vi "Read Instrument Descriptor.vi"(8 "error in (no error)":errorcluster, 11 "PXI 4070 in":refnum<class "PXI 4070.lvclass">) -> (0 "error out":errorcluster, 2 "Instrument Descriptor":refnum<k15>="Dev1", 3 "PXI 4070 out":refnum<class "PXI 4070.lvclass">)   [LabVIEW 2013, in "PXI 4070.lvclass"]
uses:
  PXI 4070.lvclass
  PXI 4070.lvclass/PXI 4070.ctl
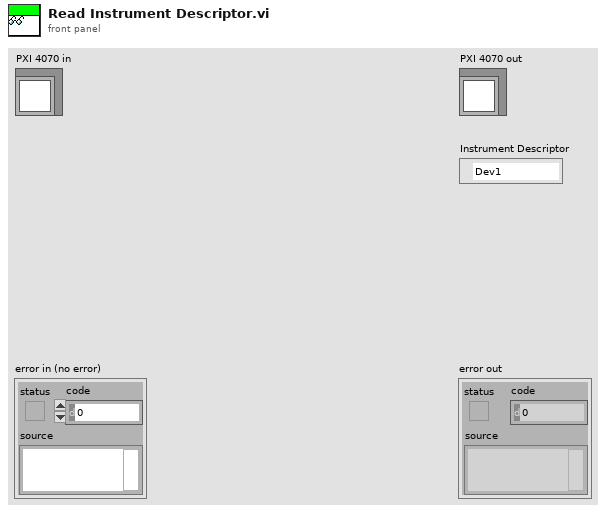
[diagram p1: front panel]
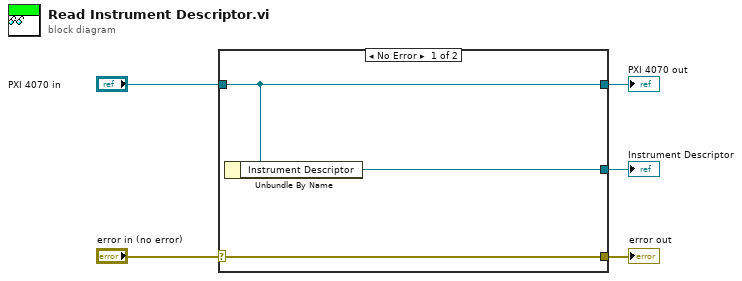
[diagram p0: block diagram]
diagram:
  n1 = case shown="No Error" "error in (no error)" {
    selector: "error in (no error)" -> [w8 w9]
    tunnel: [w8 w9] -> w4
    tunnel: [w7 w10] -> w2
    tunnel: "PXI 4070 in" -> [w7 w10]
    tunnel: [w6 _] -> w1
    frame No Error {
      n2 = Unbundle By Name(w7) -> ("Instrument Descriptor"=w6:refnum<k15>)
    }
    frame Error {
    }
  }
  "error out" <- w4
  "PXI 4070 out" <- w2
  "Instrument Descriptor" <- w1
